vi "Kinect E-Stop.vi"(1 "Reset":bool, 2 "Start Time":u32) -> (0 "Stop":bool)   [LabVIEW 2011]
doc: "Reads the Kinect 1 joystick, waiting for Button 9 (hands out to the side) to be FALSE. Crossing the driver's arms on their chest triggers the E-Stop, and stays stopped, until Reset is triggered.\n624 VI"
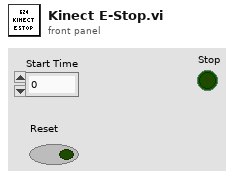
[diagram p1: front panel]
types:
  T1 = typedef "WPI_JoystickDevRef.ctl" = cluster{"Device":T2}
  T2 = typedef "WPI_JoystickDeviceEnum.ctl" = enum16{"USB 1", "USB 2", "USB 3", "USB 4", "Kinect 1", "Kinect 2"}
  T3 = typedef "WPI_JoystickButtonState.ctl" = cluster{"Button 1":bool, "Button 2":bool, "Button 3":bool, "Button 4":bool, "Button 5":bool, "Button 6":bool, "Button 7":bool, "Button 8":bool, "Button 9":bool, "Button 10":bool, "Button 11":bool, "Button 12":bool}
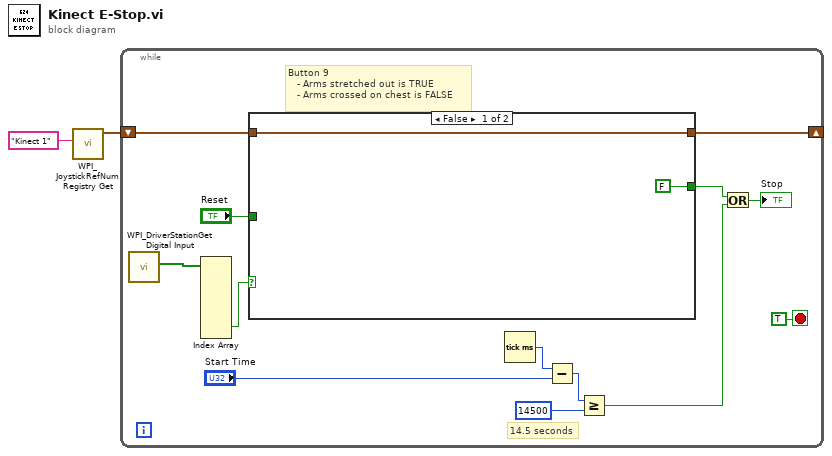
[diagram p0: block diagram]
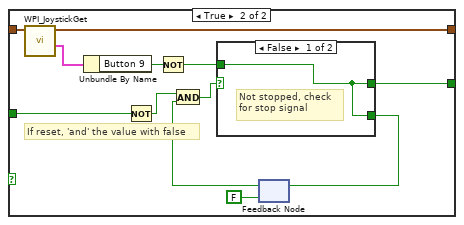
[diagram p2: hidden frame]
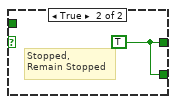
[diagram p3: hidden frame]
diagram:
  n1 = call <vilib>:"WPI_JoystickRefNum Registry Get.vi"("refnum name"="Kinect 1") -> ("JoystickDevRef"=w1:T1)  [unwired: 9 in, 1 out]
  n2 = while {
    shift-right: [w13] -> _
    shift-left: w1 -> [w15]
    stop <- TRUE stop-if-true
    # "14.5 seconds"
    # "Button 9\n   - Arms stretched out is TRUE\n   - Arms crossed on chest is FALSE"
    n3 = call <vilib>:"WPI_DriverStationGet Digital Input.vi"() -> ("Driver Station Digital Input (1-8)"=w4:bool[])  [unwired: 11 out]
    n4 = Index Array(array=w4) -> (element #7=w3:bool)  [unwired: 8 in, 7 out]
    n5 = case shown="False" w3 {
      tunnel: w15 -> [w17 w29]
      tunnel: [w17 w28] -> w13
      tunnel: "Reset" -> [_ w27]
      tunnel: [FALSE w26] -> w7
      frame False {
      }
      frame True {
        # "If reset, 'and' the value with false"
        n6 = call <vilib>:"WPI_JoystickGet.vi"("JoystickDevRef"=w29) -> ("Buttons"=w25:T3, "JoystickDevRef"=w28:T1)  [unwired: 4 in, 1 out]
        n7 = Unbundle By Name(w25) -> ("Button 9"=w24:bool)
        n8 = Not(x=w27) -> (.not. x?=w20:bool)
        n9 = Not(x=w24) -> (.not. x?=w23:bool)
        n10 = feedback #1(FALSE) -> (w19:bool)
        n11 = And(x=w20, y=w19) -> (x .and. y?=w18:bool)
        n12 = case shown="False" w18 {
          tunnel: w23 -> [w30 _]
          tunnel: [w30 w31] -> w26
          tunnel: [w30 w31] -> w21
          frame False {
            # "Not stopped, check\nfor stop signal"
          }
          frame True {
            w31 = TRUE
            # "Stopped,\nRemain Stopped"
          }
        }
        n13 = feedback-in #1(w21) -> ()
      }
    }
    n14 = Tick Count (ms)() -> (millisecond timer value=w11:u32)
    n15 = Subtract(x=w11, y="Start Time") -> (x-y=w10:u32)
    n16 = Greater Or Equal?(x=w10, y=u32 14500) -> (x >= y?=w5:bool)
    n17 = Or(x=w7, y=w5) -> (x .or. y?=→"Stop":bool)
  }
